vi "Is Message.vi"(8 "error in (no error)":errorcluster, 9 "Validation":T1, 11 "ProjectItem in":refnum<vi>) -> (0 "error out":errorcluster, 2 "Is Message":bool, 3 "ProjectItem out":refnum<vi>)   [LabVIEW 2020, in "Message Rescripter.lvlib"]
uses:
  Message Rescripter.lvlib
  MessageMakerProvider/_Message Maker/Message Maker.lvlib
  MessageMakerProvider/AFPP Shared/Validation Mode.ctl
  MessageMakerProvider/AFPP Shared/AFPP Shared.lvlib
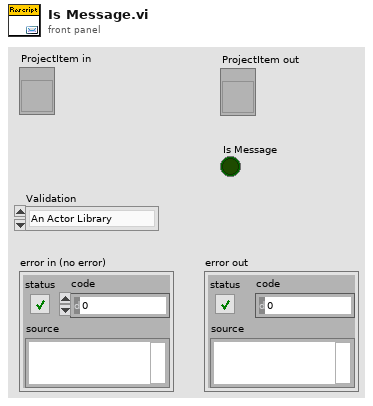
[diagram p1: front panel]
types:
  T1 = typedef "AFPP Shared.lvlib/Validation Mode.ctl" = enum16{"An Actor Library", "A Target Tag"}
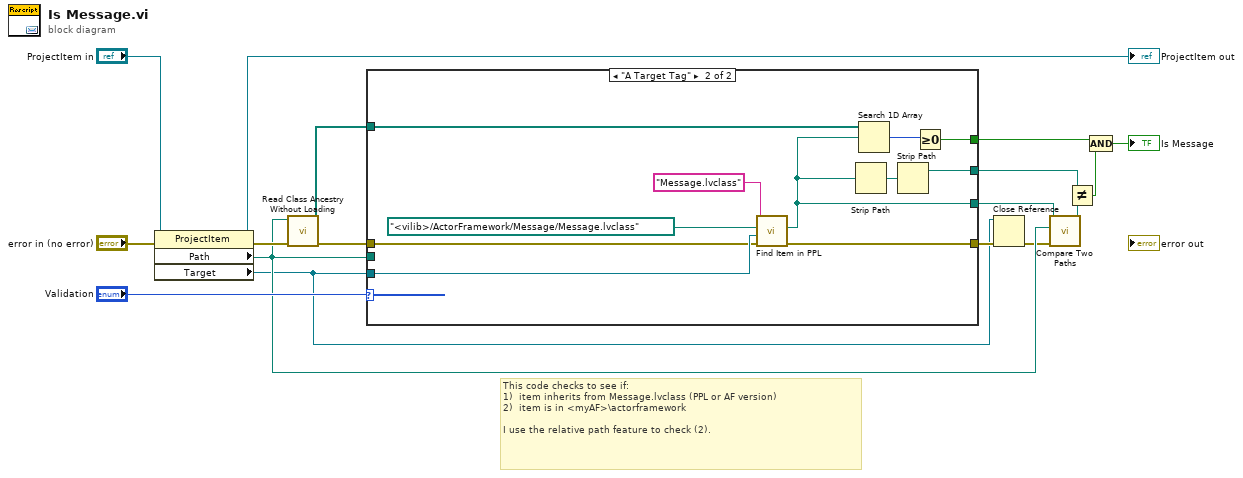
[diagram p0: block diagram]
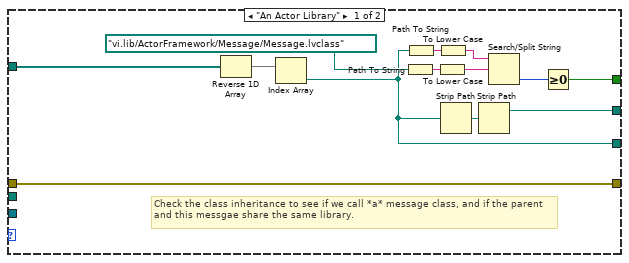
[diagram p2: hidden frame]
diagram:
  # "This code checks to see if:\n1)  item inherits from Message.lvclass (PPL or AF version)\n2)  item is in <myAF>\\actorframework\n\nI use the relative path feature to check (2)."
  n1 = property class="ProjectItem"(reference="ProjectItem in", error in="error in (no error)") -> (reference out=→"ProjectItem out":refnum<vi>, error out=w7:errorcluster, "Path"=w5:path, "Target"=w1:refnum<vi>)
  n2 = call <vilib>:"Read Class Ancestry Without Loading.vi"("error in (no error)"=w7, "LabVIEW Class Path"=w5) -> ("error out"=w6:errorcluster, "Class Ancestry"=w4:path[])  [unwired: 8 in]
  n3 = case shown="\"A Target Tag\"" "Validation" {
    tunnel: [w23 w40] -> w15
    tunnel: [w20 w39] -> w13
    tunnel: [w21 w37] -> w12
    tunnel: w6 -> [w19 w31]
    tunnel: w1 -> [_ w36]
    tunnel: w5 -> [_ _]
    tunnel: [w19 w34] -> w3
    tunnel: w4 -> [w18 w33]
    frame "An Actor Library" {
      # "Check the class inheritance to see if we call *a* message class, and if the parent and this messgae share the same library."
      n4 = Reverse 1D Array(array=w18) -> (reversed array=w25:path[])
      n5 = Index Array(array=w25) -> (element=w20:path)  [unwired: 1 in]
      n6 = Path To String(path=path "vi.lib/ActorFramework/Message/Message.lvclass") -> (string=w28:string)
      n7 = Path To String(path=w20) -> (string=w27:string)
      n8 = To Lower Case(string=w28) -> (all lower case string=w30:string)
      n9 = To Lower Case(string=w27) -> (all lower case string=w29:string)
      n10 = Strip Path(path=w20) -> (stripped path=w22:path)  [unwired: 1 out]
      n11 = Strip Path(path=w22) -> (stripped path=w21:path)  [unwired: 1 out]
      n12 = Search/Split String(string=w29, search string/char (-)=w30) -> (offset of match=w24:i32)  [unwired: 1 in, 2 out]
      n13 = Greater Or Equal To 0?(x=w24) -> (x >= 0?=w23:bool)
    }
    frame "A Target Tag" {
      n14 = call "Find Item in PPL.vi"("error in (no error)"=w31, "Target"=w36, "default path"=path "<vilib>/ActorFramework/Message/Message.lvclass" ("Path"), "qualified name"="Message.lvclass" ("key")) -> ("error out"=w34:errorcluster, "item path out"=w39:path)  [unwired: 5 in, 1 out]
      n15 = Strip Path(path=w39) -> (stripped path=w38:path)  [unwired: 1 out]
      n16 = Search 1D Array(1D array=w33, element=w39) -> (index of element=w41:i32)  [unwired: 1 in]
      n17 = Strip Path(path=w38) -> (stripped path=w37:path)  [unwired: 1 out]
      n18 = Greater Or Equal To 0?(x=w41) -> (x >= 0?=w40:bool)
    }
  }
  n19 = Close Reference(reference=w1, error in (no error)=w3) -> (error out=w2:errorcluster)
  n20 = call <vilib>:"Compare Two Paths.vi"("error in (no error)"=w2, "Path 2"=w5, "Path 1"=w13) -> ("Common Path"=w11:path)  [unwired: 5 in, 3 out]
  n21 = Not Equal?(x=w12, y=w11) -> (x != y?=w9:bool)
  n22 = Compound Arithmetic op=AND(w15, w9) -> (→"Is Message":bool)
